vi "Page_Registry_Read.vi"(6 "ctlReferences":T1, 8 "error in (no error)":errorcluster, 11 "Class in":refnum<class "IB_MSI.lvclass">) -> (0 "error out":errorcluster)   [LabVIEW 2020, in "IB_MSI.lvclass"]
uses:
  <vilib>/AppBuilder/IB_Classes/MSI/IB_MSI.lvclass
  <vilib>/AppBuilder/IB_Classes/MSI/IB_MSI.lvclass/IB_MSI.ctl
  <resource>/Framework/Providers/Builds/Installer/controls/IB_Tree_DefaultSymbols.ctl
  <vilib>/AppBuilder/IB_Classes/RegDest/IB_RegDest.lvclass
  <resource>/Framework/Providers/Builds/Installer/CDK_sTypeDef_NewFolder.ctl
  <resource>/Framework/Providers/Builds/Installer/CDK_sTypeDef_Remove.ctl
  <resource>/Framework/Providers/Builds/Installer/CDK_sTypeDef_Add.ctl
  <resource>/Framework/Providers/Builds/Installer/Pages/controls/IB_UI_Page_Registry_References.ctl
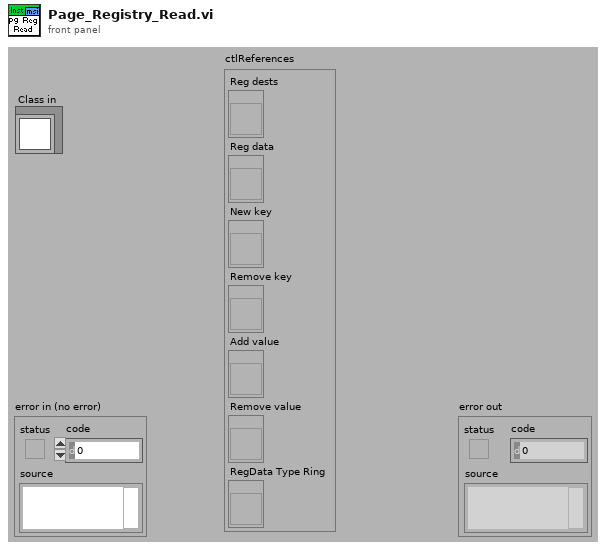
[diagram p1: front panel]
types:
  T1 = typedef "IB_UI_Page_Registry_References.ctl" = cluster{"Reg dests":refnum<vi>, "Reg data":refnum<vi>, "New key":refnum<vi>, "Remove key":refnum<vi>, "Add value":refnum<vi>, "Remove value":refnum<vi>, "RegData Type Ring":refnum<vi>}
  T2 = cluster{"Left Cell String":string, "Child Text":string[], "Child Tag":string, "Item Indent":i32, "Child Only?":bool, "Glyph Index":i32}[]
  T3 = typedef "IB_Tree_DefaultSymbols.ctl" = enum16{"<unknown>", "closed folder", "open folder", "closed folder (default)", "open folder (default)", "closed sync folder", "open sync folder", "container folder", "my computer", "build specs", "exe", "dll", "source dist", "restful web service", ".net", "packed library", "c-generator", "target"}
  T4 = cluster{"Left Cell String":string, "Child Text":string[], "Child Tag":string, "Item Indent":i32, "Child Only?":bool, "Glyph Index":i32}
  T5 = typedef "IB_RegDest.ctl" = cluster{"parentTag":string, "dirTag":string, "dirName":string, "unlock":bool, "path":string, "regData":refnum<class "IB_RegData.lvclass">[]}
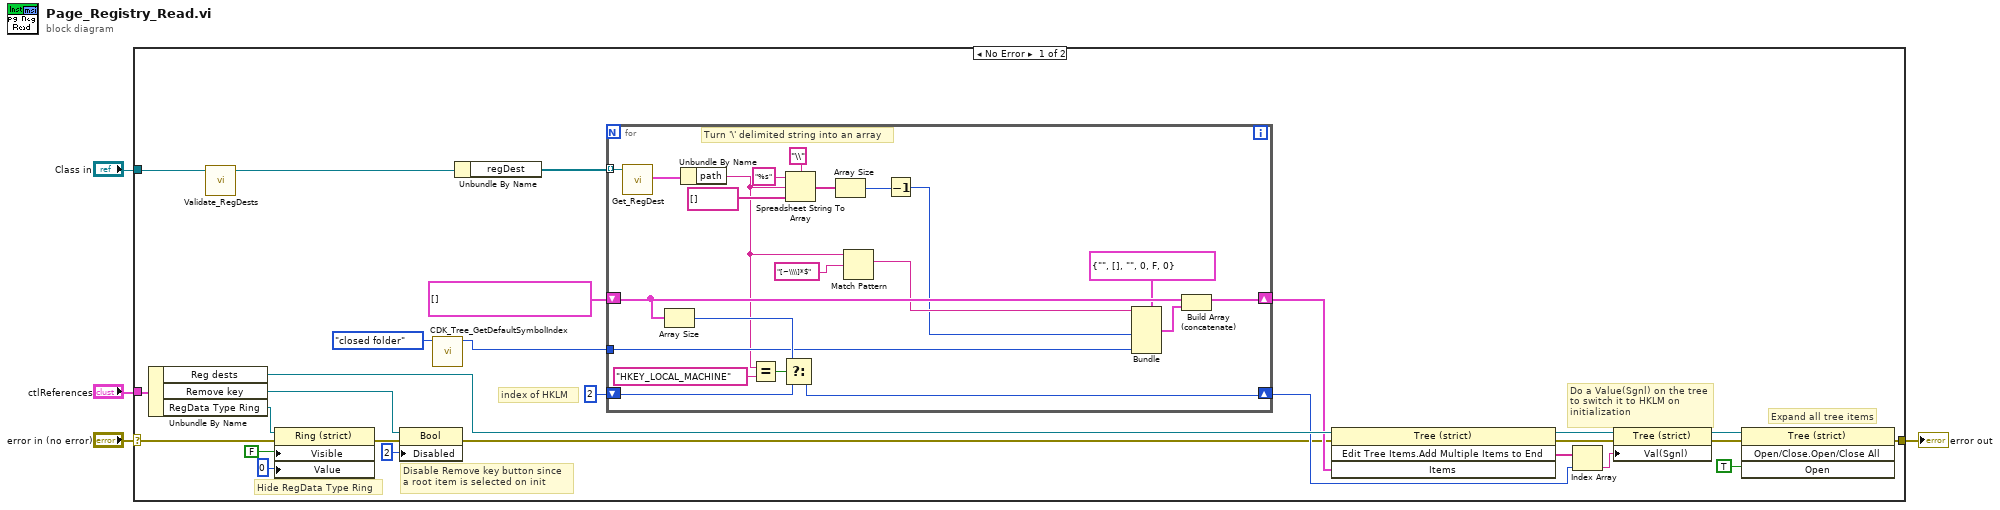
[diagram p0: block diagram]
diagram:
  n1 = case shown="No Error" "error in (no error)" {
    selector: "error in (no error)" -> [w15 w53]
    tunnel: [w19 w53] -> w3
    tunnel: "Class in" -> [w8 _]
    tunnel: "ctlReferences" -> [w31 _]
    frame No Error {
      # "index of HKLM"
      # "Disable Remove key button since\na root item is selected on init"
      # "Hide RegData Type Ring"
      # "Expand all tree items"
      # "Do a Value(Sgnl) on the tree\nto switch it to HKLM on\ninitialization"
      n2 = Unbundle By Name(w31) -> ("Reg dests"=w30:refnum<vi>, "Remove key"=w18:refnum<vi>, "RegData Type Ring"=w14:refnum<vi>)
      n3 = call <vilib>:"Validate_RegDests.vi"("IB_MSI in"=w8) -> ("IB_MSI out"=w5:refnum<class "IB_MSI.lvclass">)  [unwired: 1 in, 9 out]
      n4 = property class="Ring (strict)"(reference=w14, error in=w15, "Visible"=FALSE, "Value"=u16 0) -> (error out=w13:errorcluster)  [unwired: 1 out]
      n5 = property class="Bool"(reference=w18, error in=w13, "Disabled"=u8 2) -> (error out=w16:errorcluster)  [unwired: 1 out]
      n6 = call <resource>:"CDK_Tree_GetDefaultSymbolIndex.vi"("default symbol"=IB_Tree_DefaultSymbols."closed folder") -> ("symbol index"=w9:i32)  [unwired: 1 in, 9 out]
      n7 = Unbundle By Name(w5) -> ("regDest"=w24:refnum<class "IB_RegDest.lvclass">[])
      n8 = for {
        tunnel: w24 -> [w52] mode=indexing
        shift-right: [w47] -> w29
        shift-left: T2 [] ("Items") -> [w45]
        shift-right: [w41] -> w23
        shift-left: 2 -> [w42]
        tunnel: w9 -> [w40]
        # "Turn '\\' delimited string into an array"
        n9 = call <vilib>:"Get_RegDest.vi"("Class in"=w52) -> ("data"=w51:T5)  [unwired: 1 in, 9 out]
        n10 = Array Size(array=w45) -> (size(s)=w43:i32)
        n11 = Unbundle By Name(w51) -> ("path"=w38:string)
        n12 = Equal?(x=w38, y="HKEY_LOCAL_MACHINE") -> (x = y?=w44:bool)
        n13 = Select(t=w43, s=w44, f=w42) -> (s? t:f=w41:i32)
        n14 = Spreadsheet String To Array(delimiter (Tab)="\\", format string="%s", spreadsheet string=w38, array type (2D Dbl)=string[] []) -> (array=w36:string[])
        n15 = Array Size(array=w36) -> (size(s)=w35:i32)
        n16 = Match Pattern(string=w38, regular expression="[~\\\\]*$") -> (match substring=w37:string)  [unwired: 4 out]
        n17 = Decrement(x=w35) -> (x-1=w34:i32)
        n18 = Bundle(cluster=T4 {"Left Cell String"="", "Child Text"=[], "Child Tag"="", "Item Indent"=0, "Child Only?"=FALSE, "Glyph Index"=0} ("Item"), "Left Cell String"=w37, "Item Indent"=w34, "Glyph Index"=w40) -> (w32:T4)  [unwired: 3 out]
        n19 = Build Array (concatenate)(w45, w32) -> (w47:T2)
      }
      n20 = invoke class="Tree (strict)" method="Edit Tree Items.Add Multiple Items to End"(reference=w30, error in=w16, "Items"=w29) -> (reference out=w27:refnum<vi>, error out=w28:errorcluster, "Edit Tree Items:Add Multiple Items to End"=w26:string[])  [unwired: 1 in, 1 out]
      n21 = Index Array(array=w26, index=w23) -> (element=w25:string)
      n22 = property class="Tree (strict)"(reference=w27, error in=w28, "Val(Sgnl)"=w25) -> (reference out=w22:refnum<vi>, error out=w21:errorcluster)
      n23 = invoke class="Tree (strict)" method="Open/Close.Open/Close All"(reference=w22, error in=w21, "Open"=TRUE ("Open?")) -> (error out=w19:errorcluster)  [unwired: 1 in, 3 out]
    }
    frame Error {
    }
  }
  "error out" <- w3
